vi "Get Node.vi"(8 "error in (no error)":errorcluster, 10 "name":string, 11 "map reference in":refnum<data-value>) -> (0 "error out":errorcluster, 1 "found":bool, 2 "coordinates":dbl[](array[numeric]), 3 "map reference out":refnum<data-value>)   [LabVIEW 2017, in "NI_Robotics_DirectedGraphWorldMap.lvclass"]
doc: "Returns the coordinates of a map node in <B>map reference in</B>. You can use this VI to verify that a particular node exists or to return node <B>coordinates</B> you can plot."
uses:
  <vilib>/robotics/Navigation/shared/WorldMap/DirectedGraphWorldMap/NI_Robotics_DirectedGraphWorldMap.lvclass
  <vilib>/robotics/Navigation/shared/MapNode/DirectedGraphMapNode/NI_Robotics_DirectedGraphMapNode.lvclass
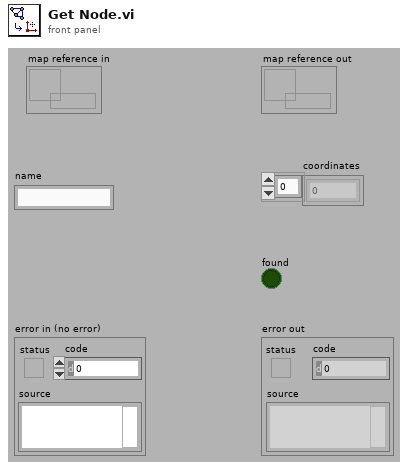
[diagram p1: front panel]
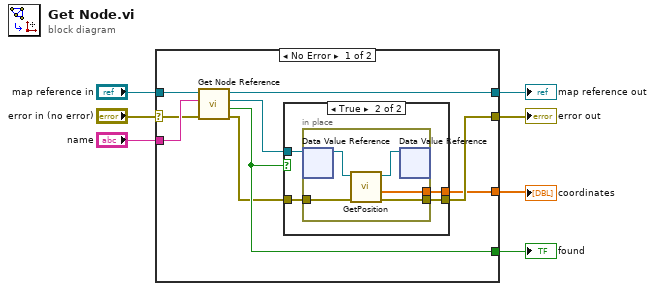
[diagram p0: block diagram]
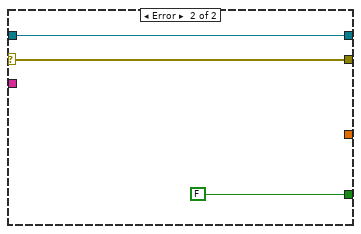
[diagram p3: hidden frame]
diagram:
  n1 = case shown="No Error" "error in (no error)" {
    selector: "error in (no error)" -> [w14 w29]
    tunnel: [w13 w29] -> w6
    tunnel: "name" -> [w16 _]
    tunnel: [w15 FALSE ("Found")] -> w4
    tunnel: [w12 _] -> w3
    tunnel: "map reference in" -> [w9 w27]
    tunnel: [w8 w27] -> w1
    frame No Error {
      n2 = call <vilib>:"Get Node Reference.vi"("error in (no error)"=w14, "name"=w16, "map reference in"=w9) -> ("error out"=w10:errorcluster, "found?"=w15:bool, "node reference"=w11:refnum<data-value>, "map reference out"=w8:refnum<data-value>)  [unwired: 5 in]
      n3 = case shown="True" w15 {
        tunnel: w11 -> [_ w21]
        tunnel: w10 -> [w17 w20]
        tunnel: [w17 w19] -> w13
        tunnel: [_ w18] -> w12
        frame False {
        }
        frame True {
          n4 = in-place {
            in-place-border: w20 -> [w24]
            in-place-border: [w23] -> w19
            in-place-border: [w22] -> w18
            n5 = in-place-dvr #1(w21) -> (w26:refnum<class "NI_Robotics_DirectedGraphMapNode.lvclass">)  [unwired: 1 out]
            n6 = call <vilib>:"GetPosition.vi"("error in (no error)"=w24, "DirectedGraphMapNode in"=w26) -> ("error out"=w23:errorcluster, "coordinates"=w22:dbl[], "DirectedGraphMapNode out"=w25:refnum<class "NI_Robotics_DirectedGraphMapNode.lvclass">)  [unwired: 6 in, 1 out]
            n7 = in-place-dvr #1(w25) -> ()  [unwired: 2 out]
          }
        }
      }
    }
    frame Error {
    }
  }
  "error out" <- w6
  "coordinates" <- w3
  "found" <- w4
  "map reference out" <- w1
